vi "Check Time in Hours.vi"() -> ()   [LabVIEW 2010]
panel:
  in  "Time Target":dbl=43200.0 format="%<%H:%M:%S>t"
  out "current time":timestamp
  out "TS Read from File":timestamp
  out "Read from File":string
  in  "File Read":path
  out "Write":string
  out "Self test not been excuted with 12 hrs":bool
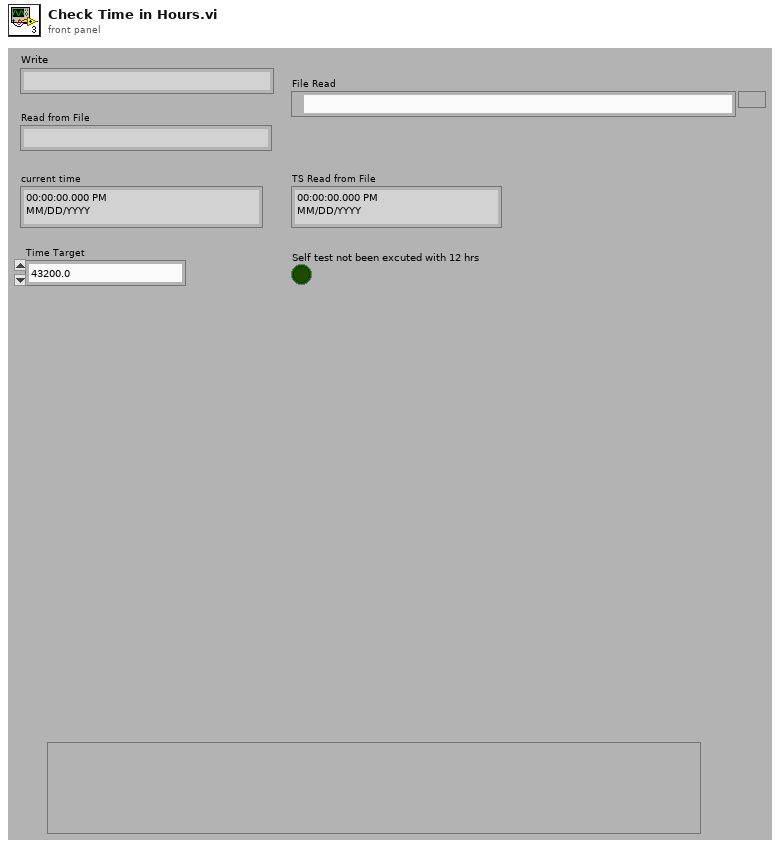
[diagram p1: front panel]
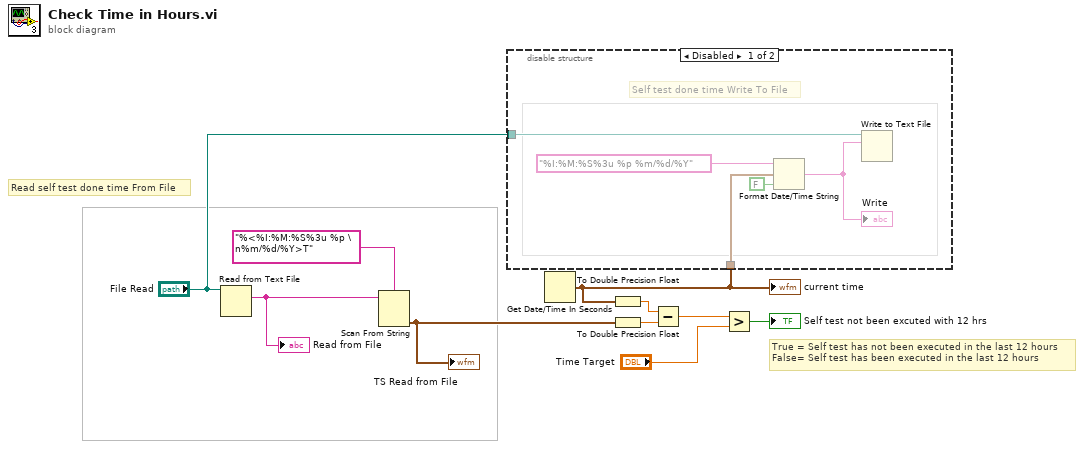
[diagram p0: block diagram]
diagram:
  # "True = Self test has not been executed in the last 12 hours\nFalse= Self test has been executed in the last 12 hours"
  # "Read self test done time From File"
  n1 = Read from Text File(file (use dialog)="File Read") -> (text=w9:string)  [unwired: 3 in, 3 out]
  "Read from File" <- w9
  n2 = Scan From String(format string="%<%I:%M:%S%3u %p \n%m/%d/%Y>T" ("time format string (%c)"), input string=w9) -> (output 1=w1:timestamp)  [unwired: 3 in, 3 out]
  "TS Read from File" <- w1
  n3 = Get Date/Time In Seconds() -> (seconds since 1Jan1904=w2:timestamp)
  "current time" <- w2
  n4 = disable-structure shown="Disabled" {
    disable-tunnel: "File Read" -> [w15 _]
    disable-tunnel: w2 -> [w14 _]
    frame Disabled {
      # "Self test done time Write To File"
      n5 = Format Date/Time String(time format string (%c)="%I:%M:%S%3u %p %m/%d/%Y", seconds (now)=w14, UTC format=FALSE) -> (date/time string=w12:string)
      "Write" <- w12
      n6 = Write to Text File(file (use dialog)=w15, text=w12) -> ()  [unwired: 2 in, 3 out]
    }
    frame Enabled {
    }
  }
  n7 = To Double Precision Float(number=w2) -> (double precision float=w7:dbl)
  n8 = To Double Precision Float(number=w1) -> (double precision float=w6:dbl)
  n9 = Subtract(x=w7, y=w6) -> (x-y=w5:dbl)
  n10 = Greater?(x=w5, y="Time Target") -> (0:→"Self test not been excuted with 12 hrs":bool)
